vi "GetBlockDiagram.vi"(6 "error in":errorcluster, 9 "VI Interpreter in":refnum<class "VI Interpreter.lvclass">) -> (0 "error out":errorcluster, 3 "VI Interpreter out":refnum<class "VI Interpreter.lvclass">, 4 "TopLevelDiagram":refnum<class "TopLevelDiagram.lvclass">)   [LabVIEW 2014, in "VI Interpreter.lvclass"]
uses:
  VI Interpreter.lvclass
  TopLevelDiagram/TopLevelDiagram.lvclass
  VI Interpreter.lvclass/VI Interpreter.ctl
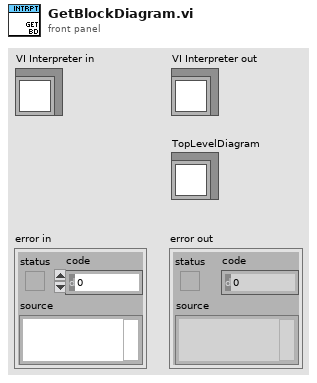
[diagram p1: front panel]
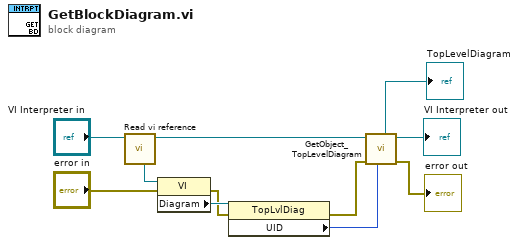
[diagram p0: block diagram]
diagram:
  n1 = call "Read vi reference.vi"("VI Interpreter in"="VI Interpreter in") -> ("VI Interpreter out"=w6:refnum<class "VI Interpreter.lvclass">, "vi reference"=w10:refnum<vi>)  [unwired: 7 in]
  n2 = property class="VI"(reference=w10, error in="error in") -> (error out=w7:errorcluster, "Diagram"=w8:refnum<vi>)  [unwired: 1 out]
  n3 = property class="TopLvlDiag"(reference=w8, error in=w7) -> (error out=w4:errorcluster, "UID"=w5:i32)  [unwired: 1 out]
  n4 = call "GetObject_TopLevelDiagram.vi"("UID"=w5, "error in"=w4, "VI Interpreter in"=w6) -> ("error out"=→"error out":errorcluster, "VI Interpreter out"=→"VI Interpreter out":refnum<class "VI Interpreter.lvclass">, "TopLevelDiagram"=→"TopLevelDiagram":refnum<class "TopLevelDiagram.lvclass">)  [unwired: 3 in, 1 out]
